vi "Set DVA Info wrapper.vi"(7 "bAckEna":i32, 8 "error in (no error)":errorcluster caption="错误输入（无错误）", 9 "DVA_INFO_OBJ In":T1, 10 "dwCanNodeId":u32, 11 "dwDevIndex":u32) -> (0 "error out":errorcluster caption="错误输出", 1 "DVA_INFO_OBJ Out":T1, 3 "function return":u32)   [LabVIEW 2016, in "UISimCanFunc_wrapper.lvlib"]
doc: "_declspec (dllexport) DWORD SetDVAInfo_wrapper(DWORD dwDevIndex, DWORD dwCanNodeId,\n P_DUMMY_DVA_INFO_OBJ pDummyDvaInfoIn, BOOL bAckEna, P_DUMMY_DVA_INFO_OBJ pDummyDvaInfoOut);"
uses:
  <userlib>/UISimCanFunc_wrapper/UISimCanFunc_wrapper.lvlib
  <userlib>/UISimCanFunc_wrapper/ctl/DVA_INFO_OBJ.ctl
  <userlib>/UISimCanFunc_wrapper/UISimCanFunc_wrapper.dll
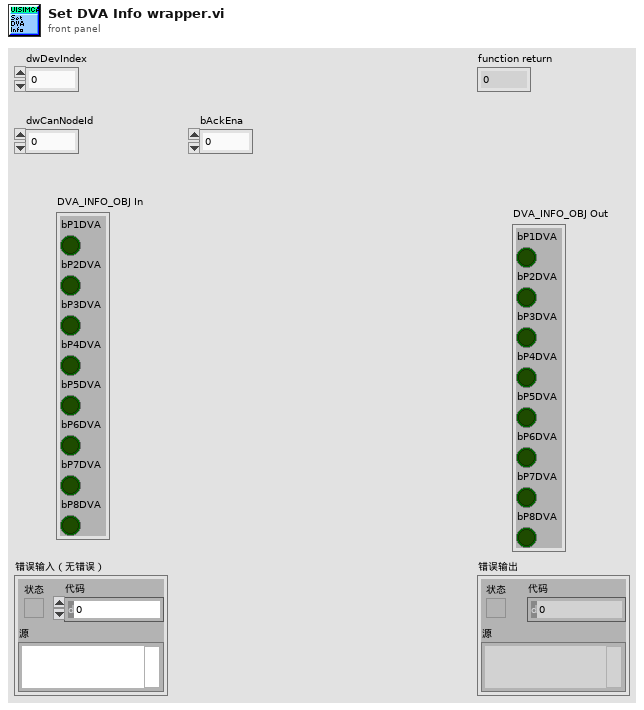
[diagram p1: front panel]
types:
  T1 = typedef "UISimCanFunc_wrapper.lvlib/DVA_INFO_OBJ.ctl" = cluster{"bP1DVA":bool, "bP2DVA":bool, "bP3DVA":bool, "bP4DVA":bool, "bP5DVA":bool, "bP6DVA":bool, "bP7DVA":bool, "bP8DVA":bool}
  T2 = cluster{"bP1DVA":i32, "bP2DVA":i32, "bP3DVA":i32, "bP4DVA":i32, "bP5DVA":i32, "bP6DVA":i32, "bP7DVA":i32, "bP8DVA":i32}
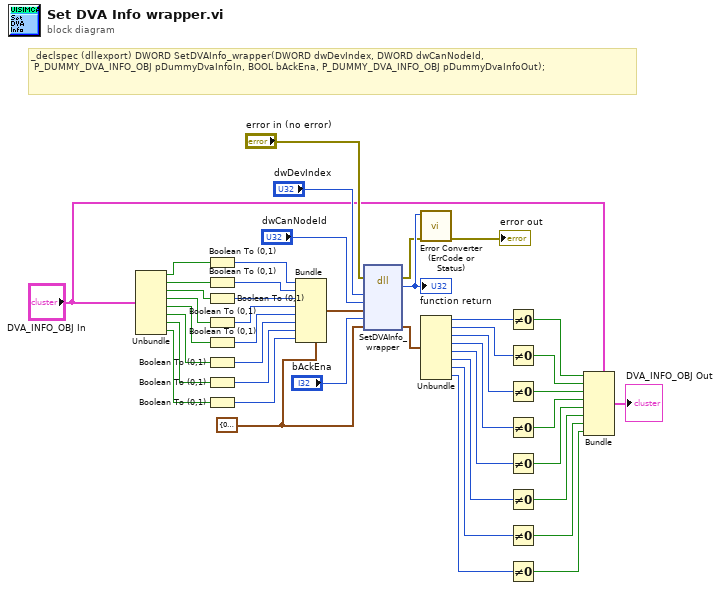
[diagram p0: block diagram]
diagram:
  w20 = T2 {"bP1DVA"=0, "bP2DVA"=0, "bP3DVA"=0, "bP4DVA"=0, "bP5DVA"=0, "bP6DVA"=0, "bP7DVA"=0, "bP8DVA"=0} ("pDummyDvaInfoIn")
  # "_declspec (dllexport) DWORD SetDVAInfo_wrapper(DWORD dwDevIndex, DWORD dwCanNodeId,\n\tP_DUMMY_DVA_INFO_OBJ pDummyDvaInfoIn, BOOL bAckEna, P_DUMMY_DVA_INFO_OBJ pDummyDvaInfoOut);"
  n1 = Unbundle("DVA_INFO_OBJ In") -> ("bP1DVA"=w37:bool, "bP2DVA"=w36:bool, "bP3DVA"=w35:bool, "bP4DVA"=w34:bool, "bP5DVA"=w33:bool, "bP6DVA"=w32:bool, "bP7DVA"=w31:bool, "bP8DVA"=w30:bool)
  n2 = Boolean To (0,1)(Boolean=w37) -> (0, 1=w29:i16)
  n3 = Boolean To (0,1)(Boolean=w36) -> (0, 1=w28:i16)
  n4 = Boolean To (0,1)(Boolean=w35) -> (0, 1=w27:i16)
  n5 = Boolean To (0,1)(Boolean=w34) -> (0, 1=w26:i16)
  n6 = Boolean To (0,1)(Boolean=w33) -> (0, 1=w25:i16)
  n7 = Boolean To (0,1)(Boolean=w32) -> (0, 1=w24:i16)
  n8 = Boolean To (0,1)(Boolean=w31) -> (0, 1=w23:i16)
  n9 = Boolean To (0,1)(Boolean=w30) -> (0, 1=w22:i16)
  n10 = Bundle(cluster=w20, "bP1DVA"=w29, "bP2DVA"=w28, "bP3DVA"=w27, "bP4DVA"=w26, "bP5DVA"=w25, "bP6DVA"=w24, "bP7DVA"=w23, "bP8DVA"=w22) -> (w21:T2)
  n11 = dll-call lib="C:/Program Files (x86)/National Instruments/LabVIEW 2016/user.lib/UISimCanFunc_wrapper/UISimCanFunc_wrapper.*" fn="SetDVAInfo_wrapper"(error in="error in (no error)", "dwDevIndex"="dwDevIndex", "dwCanNodeId"="dwCanNodeId", "pDummyDvaInfoIn"=w21, "bAckEna"="bAckEna", "pDummyDvaInfoOut"=w20) -> (error out=w39:errorcluster, w44:u32, "pDummyDvaInfoOut"=w19:T2)  [unwired: 6 in, 1 out]
  "function return" <- w44
  n12 = call <userlib>:"Error Converter (ErrCode or Status).vi"("error in (no error)"=w39, "error code"=w44) -> ("error out"=→"error out":errorcluster)  [unwired: 9 in]
  n13 = Unbundle(w19) -> ("bP1DVA"=w16:i32, "bP2DVA"=w15:i32, "bP3DVA"=w14:i32, "bP4DVA"=w13:i32, "bP5DVA"=w12:i32, "bP6DVA"=w11:i32, "bP7DVA"=w10:i32, "bP8DVA"=w9:i32)
  n14 = Not Equal To 0?(x=w16) -> (x != 0?=w8:bool)
  n15 = Not Equal To 0?(x=w15) -> (x != 0?=w7:bool)
  n16 = Not Equal To 0?(x=w14) -> (x != 0?=w6:bool)
  n17 = Not Equal To 0?(x=w13) -> (x != 0?=w5:bool)
  n18 = Not Equal To 0?(x=w12) -> (x != 0?=w4:bool)
  n19 = Not Equal To 0?(x=w11) -> (x != 0?=w3:bool)
  n20 = Not Equal To 0?(x=w10) -> (x != 0?=w2:bool)
  n21 = Not Equal To 0?(x=w9) -> (x != 0?=w1:bool)
  n22 = Bundle(cluster="DVA_INFO_OBJ In", "bP1DVA"=w8, "bP2DVA"=w7, "bP3DVA"=w6, "bP4DVA"=w5, "bP5DVA"=w4, "bP6DVA"=w3, "bP7DVA"=w2, "bP8DVA"=w1) -> (→"DVA_INFO_OBJ Out":T1)
